vi "2D Compass Plot.vi"() -> ()   [LabVIEW 2017, in "2D_Merge.lvlib"]
uses:
  <vilib>/Math Plots/2D Math Plots/Merge VIs/2D_Merge.lvlib
  <vilib>/Math Plots/2D Math Plots/2D Compass/2D Compass XCtrl/2D Compass.xctl
  <vilib>/Math Plots/2D Math Plots/2D Compass/2D Compass Datatype/Public/Plot Helper (Vector).vi
  <vilib>/Math Plots/2D Math Plots/2D Compass/2D Compass Datatype/2D Compass Datatype.lvclass
panel:
  out "2D Compass":refnum<class "2D Plot Datatype.lvclass">[](xcontrol)
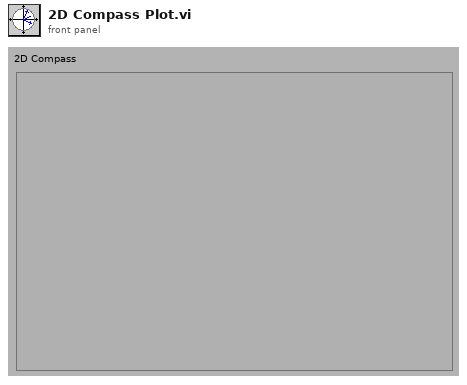
[diagram p1: front panel]
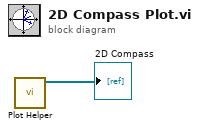
[diagram p0: block diagram]
diagram:
  n1 = call-poly <vilib>:"Plot Helper.vi"() -> ("2D Plot Class Obj Array out"=→"2D Compass":refnum<class "2D Plot Datatype.lvclass">[])  [unwired: 4 in, 7 out]
